vi "WLAN Rx Test Get Default USL.vi"(8 "error in (no error)":errorcluster, 11 "Template Rx Test in":refnum<class "niDTS WLAN Rx Test.lvclass">) -> (0 "error out":errorcluster, 2 "Default USL":T1, 3 "Template Rx Test out":refnum<class "niDTS WLAN Rx Test.lvclass">)   [LabVIEW 2015, in "niDTS WLAN.lvlib" / "niDTS WLAN Rx Test.lvclass"]
uses:
  niDTS WLAN Rx Test.lvclass
  Includes/niDTS WLAN Rx Test INC Results.ctl
  niDTS WLAN Rx Test.lvclass/niDTS WLAN Rx Test.ctl
  niDTS WLAN.lvlib
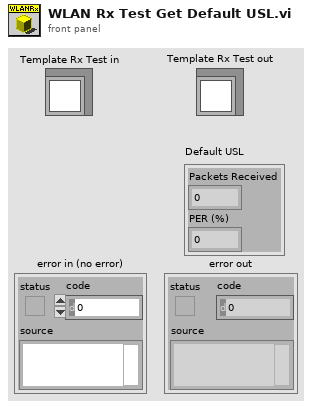
[diagram p1: front panel]
types:
  T1 = typedef "niDTS WLAN.lvlib/niDTS WLAN Rx Test INC Results.ctl" = cluster{"Packets Received":i32, "PER (%)":dbl}
  T2 = typedef "niDTS WLAN.lvlib/niDTS WLAN INC Standard.ctl" = enum16{"802.11 b DSSS", "802.11 a/g OFDM", "802.11 n HT", "802.11 ac VHT"}
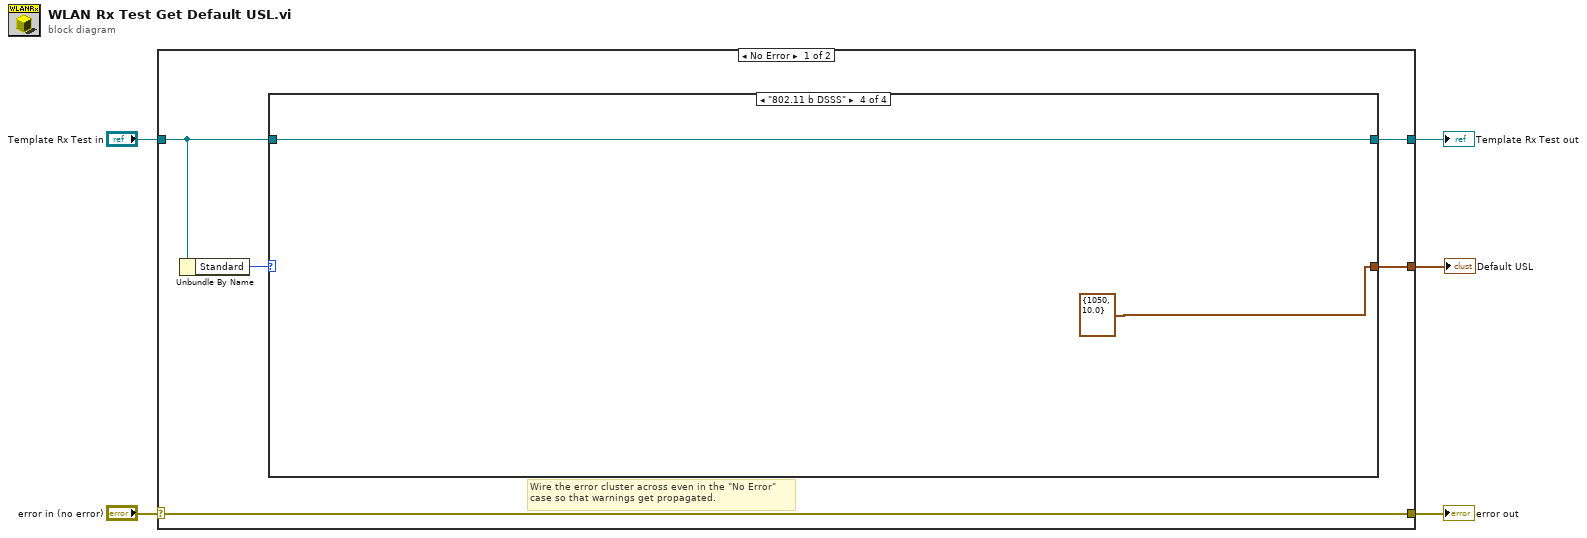
[diagram p0: block diagram]
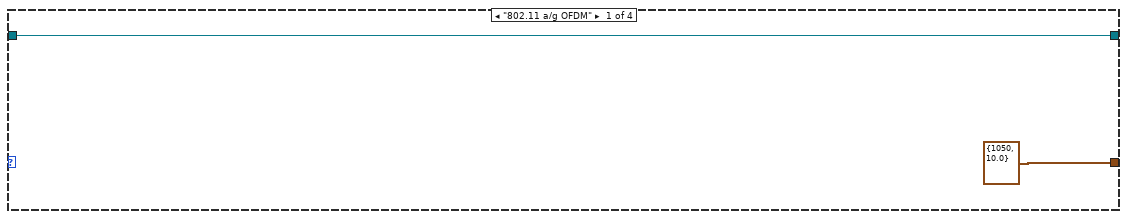
[diagram p2: hidden frame]
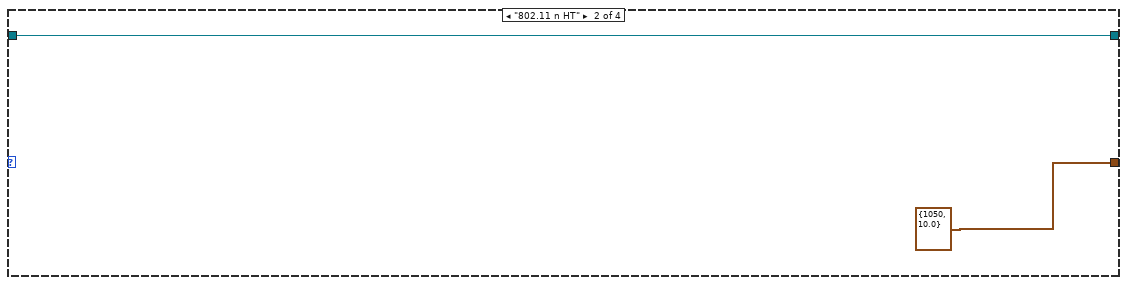
[diagram p3: hidden frame]
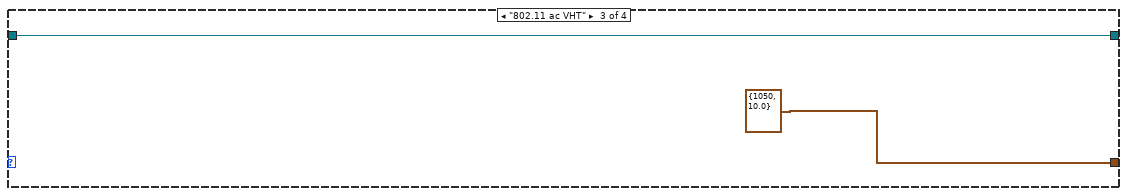
[diagram p4: hidden frame]
diagram:
  n1 = case shown="No Error" "error in (no error)" {
    selector: "error in (no error)" -> [w10 w20]
    tunnel: [w10 w20] -> w2
    tunnel: [w7 w19] -> w4
    tunnel: "Template Rx Test in" -> [w8 w19]
    tunnel: [w6 _] -> w1
    frame No Error {
      # "Wire the error cluster across even in the \"No Error\"\ncase so that warnings get propagated."
      n2 = Unbundle By Name(w8) -> ("Standard"=w9:T2)
      n3 = case shown="\"802.11 b DSSS\"" w9 {
        tunnel: w8 -> [w12 w14 w16 w18]
        tunnel: [w12 w14 w16 w18] -> w7
        tunnel: [T1 {"Packets Received"=1050, "PER (%)"=10.0} ("Default USL") T1 {"Packets Received"=1050, "PER (%)"=10.0} ("Default USL") T1 {"Packets Received"=1050, "PER (%)"=10.0} ("Default USL") T1 {"Packets Received"=1050, "PER (%)"=10.0} ("Default USL")] -> w6
        frame "802.11 a/g OFDM" {
        }
        frame "802.11 n HT" {
        }
        frame "802.11 ac VHT" {
        }
        frame "802.11 b DSSS" {
        }
      }
    }
    frame Error {
    }
  }
  "error out" <- w2
  "Template Rx Test out" <- w4
  "Default USL" <- w1
